vi "Connect.vi"(8 "error in (no error)":errorcluster, 11 "UR5 Robot in":refnum<class "UR5 Robot.lvclass">) -> (0 "error out":errorcluster, 3 "UR5 Robot out":refnum<class "UR5 Robot.lvclass">)   [LabVIEW 2018, in "UR5 Robot.lvlib" / "UR5 Robot.lvclass"]
uses:
  UR5 Robot.lvclass
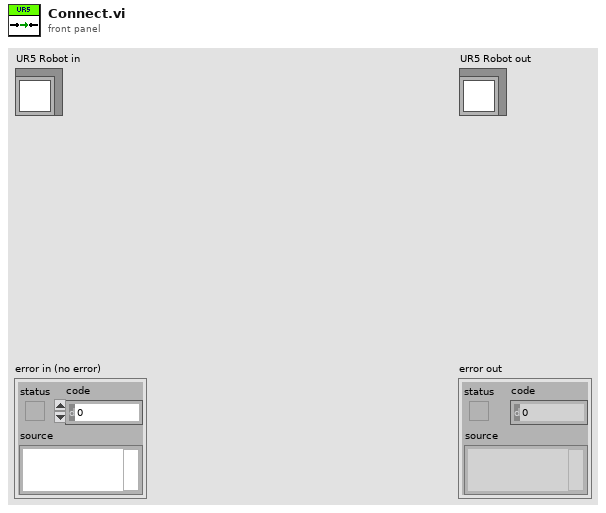
[diagram p1: front panel]
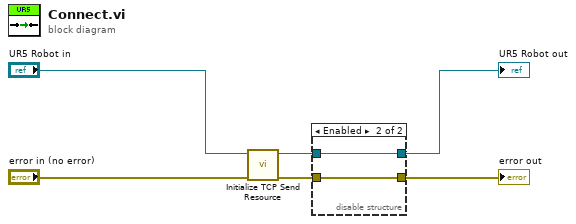
[diagram p0: block diagram]
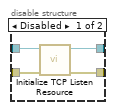
[diagram p2: hidden frame]
diagram:
  n1 = call "Initialize TCP Send Resource.vi"("error in (no error)"="error in (no error)", "UR5 Robot in"="UR5 Robot in") -> ("error out"=w3:errorcluster, "UR5 Robot out"=w4:refnum<class "UR5 Robot.lvclass">)  [unwired: 8 in]
  n2 = disable-structure shown="Enabled" {
    disable-tunnel: w4 -> [w10 w12]
    disable-tunnel: w3 -> [w9 w11]
    disable-tunnel: [w8 w11] -> w2
    disable-tunnel: [w7 w12] -> w1
    frame Disabled {
      n3 = call "Initialize TCP Listen Resource.vi"("error in (no error)"=w9, "UR5 Robot in"=w10) -> ("error out"=w8:errorcluster, "UR5 Robot out"=w7:refnum<class "UR5 Robot.lvclass">)  [unwired: 8 in]
    }
    frame Enabled {
    }
  }
  "error out" <- w2
  "UR5 Robot out" <- w1
